vi "Page_Advanced_ReadAll.vi"(6 "ctl references":T1, 8 "error in (no error)":errorcluster, 10 "Calculated IncludeHWConfig":bool, 11 "AB_Build in":refnum<class "AB_Build.lvclass">) -> (0 "error out":errorcluster, 3 "AB_Build out":refnum<class "AB_Build.lvclass">)   [LabVIEW 2020, in "AB_Build.lvclass"]
uses:
  <vilib>/AppBuilder/AB_Classes/Build/AB_Build.lvclass
  <resource>/Framework/Providers/Builds/AppBuilder/AB_UI_Page_Advanced_References.ctl
  <vilib>/AppBuilder/AB_Classes/Build/AB_Build.lvclass/AB_Build.ctl
  <vilib>/AppBuilder/AB_Classes/Destination/AB_Destination.lvclass
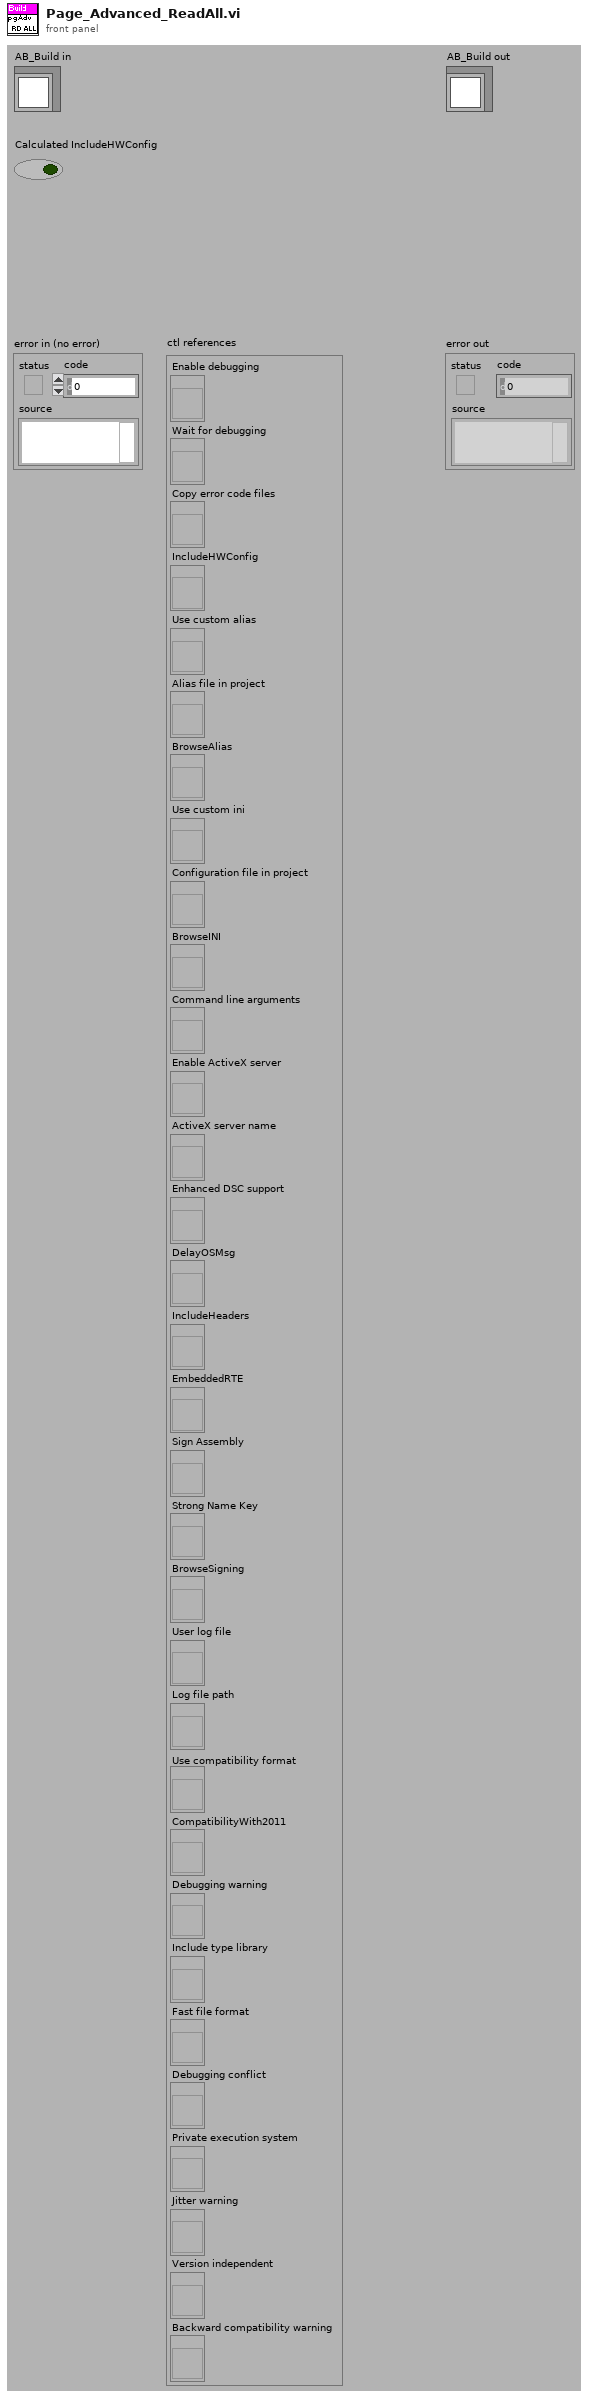
[diagram p1: front panel]
types:
  T1 = typedef "AB_UI_Page_Advanced_References.ctl" = cluster{"Enable debugging":refnum<vi>, "Wait for debugging":refnum<vi>, "Copy error code files":refnum<vi>, "IncludeHWConfig":refnum<vi>, "Use custom alias":refnum<vi>, "Alias file in project":refnum<vi>, "BrowseAlias":refnum<vi>, "Use custom ini":refnum<vi>, "Configuration file in project":refnum<vi>, "BrowseINI":refnum<vi>, "Command line arguments":refnum<vi>, "Enable ActiveX server":refnum<vi>, "ActiveX server name":refnum<vi>, "Enhanced DSC support":refnum<vi>, "DelayOSMsg":refnum<vi>, "IncludeHeaders":refnum<vi>, "EmbeddedRTE":refnum<vi>, "Sign Assembly":refnum<vi>, "Strong Name Key":refnum<vi>, "BrowseSigning":refnum<vi>, "User log file":refnum<vi>, "Log file path":refnum<vi>, "Use compatibility format":refnum<vi>, "CompatibilityWith2011":refnum<vi>, "Debugging warning":refnum<vi>, "Include type library":refnum<vi>, "Fast file format":refnum<vi>, "Debugging conflict":refnum<vi>, "Private execution system":refnum<vi>, "Jitter warning":refnum<vi>, "Version independent":refnum<vi>, "Backward compatibility warning":refnum<vi>}
  T2 = typedef "AB_Destination.ctl" = cluster{"destName":string, "path":path, "libraryName":string, "preserveHierarchy":bool, "eng_inBuild":bool, "eng_libraryReference":refnum<vi>, "eng_restictAddToNewLibrary":bool}
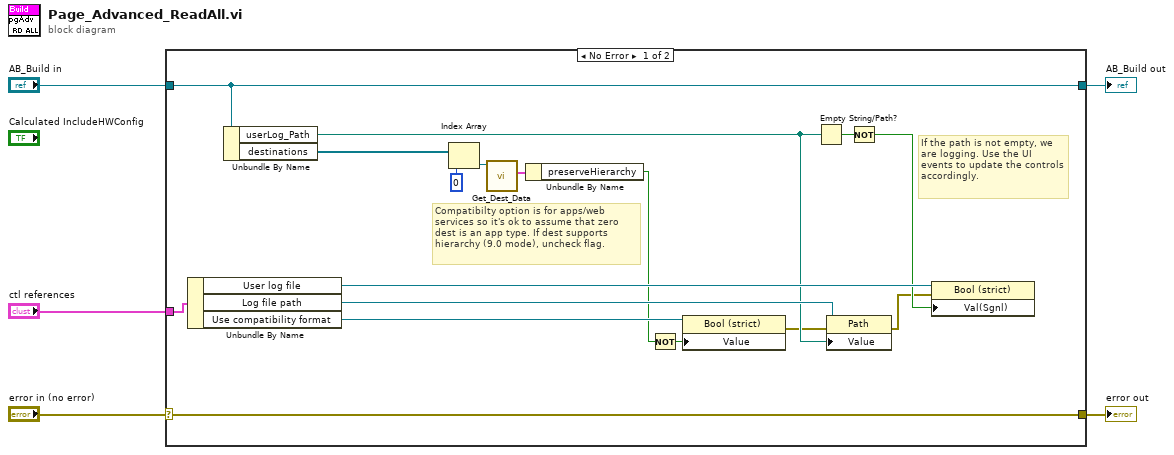
[diagram p0: block diagram]
diagram:
  n1 = case shown="No Error" "error in (no error)" {
    selector: "error in (no error)" -> [w22 w24]
    tunnel: [w22 w24] -> w4
    tunnel: [w21 w23] -> w2
    tunnel: "AB_Build in" -> [w21 w23]
    tunnel: "ctl references" -> [w20 _]
    frame No Error {
      # "Compatibilty option is for apps/web services so it's ok to assume that zero dest is an app type. If dest supports hierarchy (9.0 mode), uncheck flag."
      # "If the path is not empty, we are logging. Use the UI events to update the controls accordingly."
      n2 = Unbundle By Name(w20) -> ("User log file"=w19:refnum<vi>, "Log file path"=w16:refnum<vi>, "Use compatibility format"=w13:refnum<vi>)
      n3 = Unbundle By Name(w21) -> ("userLog_Path"=w15:path, "destinations"=w11:refnum<class "AB_Destination.lvclass">[])
      n4 = Index Array(array=w11, index=0) -> (element=w10:refnum<class "AB_Destination.lvclass">)
      n5 = call <vilib>:"Get_Dest_Data.vi"("Class in"=w10) -> ("destName"=w8:T2)  [unwired: 1 in, 9 out]
      n6 = Unbundle By Name(w8) -> ("preserveHierarchy"=w6:bool)
      n7 = Not(x=w6) -> (.not. x?=w7:bool)
      n8 = property class="Bool (strict)"(reference=w13, "Value"=w7) -> (error out=w12:errorcluster)  [unwired: 1 in, 1 out]
      n9 = Empty String/Path?(string/path=w15) -> (empty?=w18:bool)
      n10 = property class="Path"(reference=w16, error in=w12, "Value"=w15) -> (error out=w14:errorcluster)  [unwired: 1 out]
      n11 = Not(x=w18) -> (.not. x?=w17:bool)
      n12 = property class="Bool (strict)"(reference=w19, error in=w14, "Val(Sgnl)"=w17) -> ()  [unwired: 2 out]
    }
    frame Error {
    }
  }
  "error out" <- w4
  "AB_Build out" <- w2
